vi "waitForTemperature.vi"(4 "Type":enum16{"In Range", "Less", "Greater"}(ring), 6 "Channel":i32, 8 "error in (no error)":errorcluster, 9 "Tolerance (K)":dbl=0.005, 10 "Setpoint (K)":dbl, 11 "Instrument.Cryostat in":refnum<class "Instrument.Cryostat.lvclass">) -> (0 "error out":errorcluster, 3 "Instrument.Cryostat out":refnum<class "Instrument.Cryostat.lvclass">)   [LabVIEW 2019, in "Instrument.Cryostat.lvclass"]
uses:
  Instrument.Cryostat.lvclass
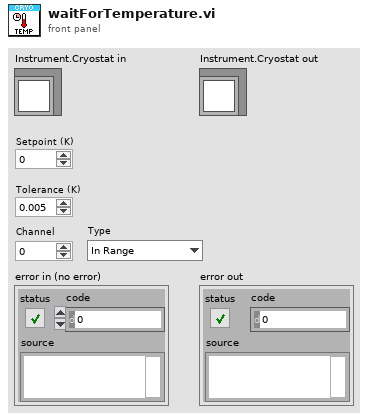
[diagram p1: front panel]
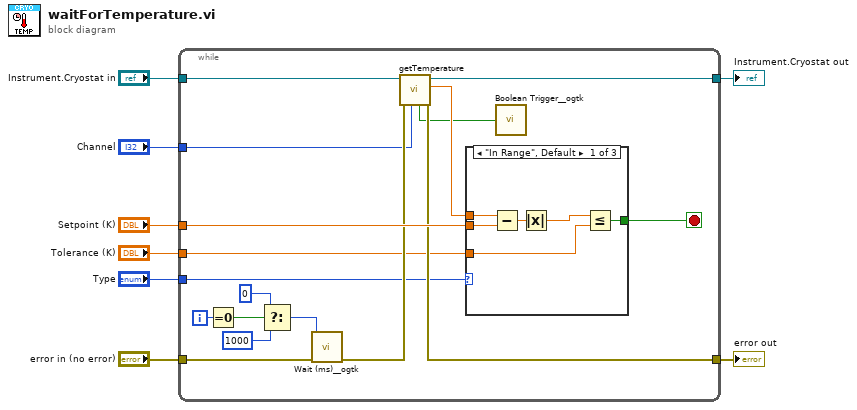
[diagram p0: block diagram]
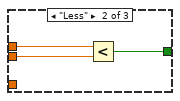
[diagram p2: hidden frame]
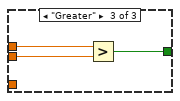
[diagram p3: hidden frame]
diagram:
  n1 = while {
    tunnel: "Setpoint (K)" -> [w25]
    tunnel: "Instrument.Cryostat in" -> [w20]
    tunnel: "error in (no error)" -> [w21]
    tunnel: [w23] -> w7
    tunnel: [w19] -> w8
    tunnel: "Channel" -> [w18]
    tunnel: "Type" -> [w17]
    tunnel: "Tolerance (K)" -> [w16]
    i -> [w14]
    stop <- w9 stop-if-true
    n2 = Equal To 0?(x=w14) -> (x = 0?=w15:bool)
    n3 = Select(t=u32 0, s=w15, f=u32 1000 ("milliseconds to wait")) -> (s? t:f=w13:u32)
    n4 = call <userlib>:"Wait (ms)__ogtk.vi"("error in (no error)"=w21, "milliseconds to wait"=w13) -> ("error out"=w24:errorcluster)  [unwired: 8 in, 1 out]
    n5 = call-dynamic "getTemperature.vi"("Channel"=w18, "error in (no error)"=w24, "Instrument.Cryostat in"=w20) -> ("error out"=w23:errorcluster, "Temperature (K)"=w22:dbl, "Instrument.Cryostat out"=w19:refnum<class "Instrument.Cryostat.lvclass">, "Finished?"=w10:bool)  [unwired: 4 in, 1 out]
    n6 = case shown="\"In Range\", Default" w17 {
      tunnel: w25 -> [w29 w34 w37]
      tunnel: [w28 w32 w35] -> w9
      tunnel: w22 -> [w27 w33 w36]
      tunnel: w16 -> [w26 _ _]
      frame "In Range", Default {
        n7 = Subtract(x=w27, y=w29) -> (x-y=w31:dbl)
        n8 = Absolute Value(x=w31) -> (abs(x)=w30:dbl)
        n9 = Less Or Equal?(x=w30, y=w26) -> (x <= y?=w28:bool)
      }
      frame "Less" {
        n10 = Less?(x=w33, y=w34) -> (x < y?=w32:bool)
      }
      frame "Greater" {
        n11 = Greater?(x=w36, y=w37) -> (0:w35:bool)
      }
    }
    n12 = call <userlib>:"Boolean Trigger__ogtk.vi"("Boolean Input"=w10) -> ()  [unwired: 1 in, 2 out]
  }
  "Instrument.Cryostat out" <- w8
  "error out" <- w7
